vi "VI.vi"(8 "error in":errorcluster, 11 "PythonConverter_GUI in":refnum<class "PythonConverter_GUI.lvclass">) -> (0 "error out":errorcluster, 3 "PythonConverter_GUI out":refnum<class "PythonConverter_GUI.lvclass">, 4 "VI":string)   [LabVIEW 2014, in "PythonConverter_GUI.lvclass"]
uses:
  PythonConverter_GUI.lvclass
  PythonConverter_GUI.lvclass/PythonConverter_GUI.ctl
  Parsing/ClassTypeTD.ctl
  Parsing/Python Functions.lvlib
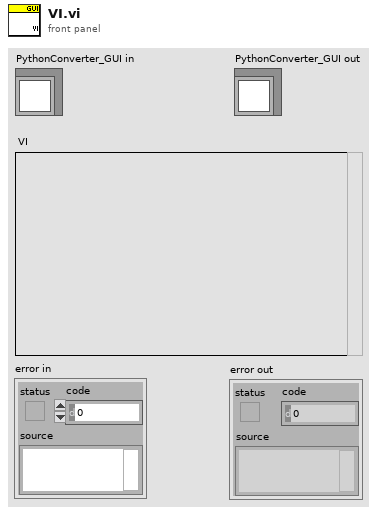
[diagram p1: front panel]
types:
  T1 = typedef "Python Functions.lvlib/ClassTypeTD.ctl" = enum16{"class", "function"}
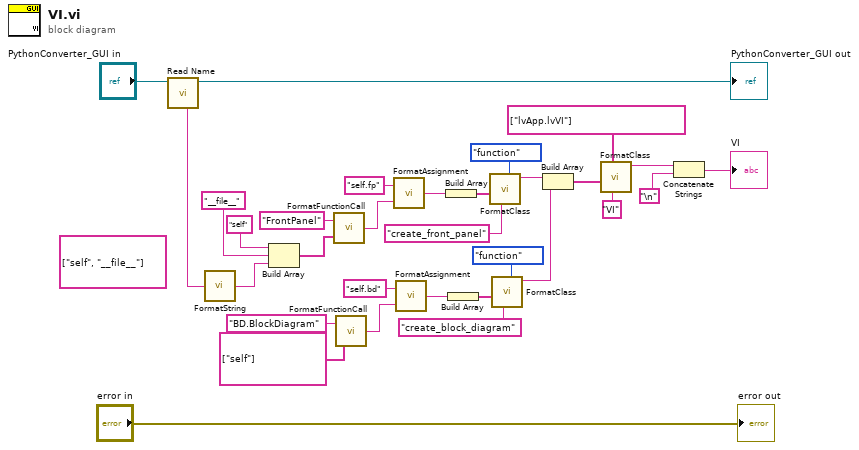
[diagram p0: block diagram]
diagram:
  (unwired) string[] ["self", "__file__"] ("parameters")
  n1 = call "Read Name.vi"("PythonConverter_GUI in"="PythonConverter_GUI in") -> ("PythonConverter_GUI out"=→"PythonConverter_GUI out":refnum<class "PythonConverter_GUI.lvclass">, "Name"=w2:string)  [unwired: 7 in]
  n2 = call "FormatString.vi"("value"=w2) -> ("python object"=w1:string)
  n3 = Build Array("self" ("String"), "__file__" ("String"), w1) -> (w4:string[])
  n4 = call "FormatFunctionCall.vi"("parameters"=w4, "function"="FrontPanel") -> ("python object"=w21:string)
  n5 = call "FormatFunctionCall.vi"("parameters"=string[] ["self"], "function"="BD.BlockDiagram") -> ("python object"=w13:string)
  n6 = call "FormatAssignment.vi"("value"=w21, "name"="self.fp") -> ("python assignment"=w19:string)
  n7 = call "FormatAssignment.vi"("value"=w13, "name"="self.bd") -> ("python assignment"=w16:string)
  n8 = Build Array(w19) -> (w18:string[])
  n9 = Build Array(w16) -> (w17:string[])
  n10 = call "FormatClass.vi"("type"=ClassTypeTD."function", "name"="create_front_panel", "body"=w18) -> ("python"=w26:string)  [unwired: 8 in]
  n11 = call "FormatClass.vi"("type"=ClassTypeTD."function", "name"="create_block_diagram", "body"=w17) -> ("python"=w9:string)  [unwired: 8 in]
  n12 = Build Array(w26, w9) -> (w25:string[])
  n13 = call "FormatClass.vi"("name"="VI", "parameters/ancestors"=string[] ["lvApp.lvVI"], "body"=w25) -> ("python"=w28:string)  [unwired: 8 in]
  n14 = Concatenate Strings(w28, "\n") -> (→"VI":string)
  "error out" <- "error in"
